vi "啮合 位移量对应扭矩.vi"(7 "目标位移量":dbl=136.0 format="%#_13g", 9 "扭矩":dbl[](array[numeric]), 11 "位移量":dbl[](array[numeric])) -> (3 "推力右扭矩":dbl)   [LabVIEW 2015, in "Logging.lvlib"]
uses:
  Logging.lvlib
panel:
  out "波形图 2":dbl[](graph)
  out "波形图":dbl[](graph)
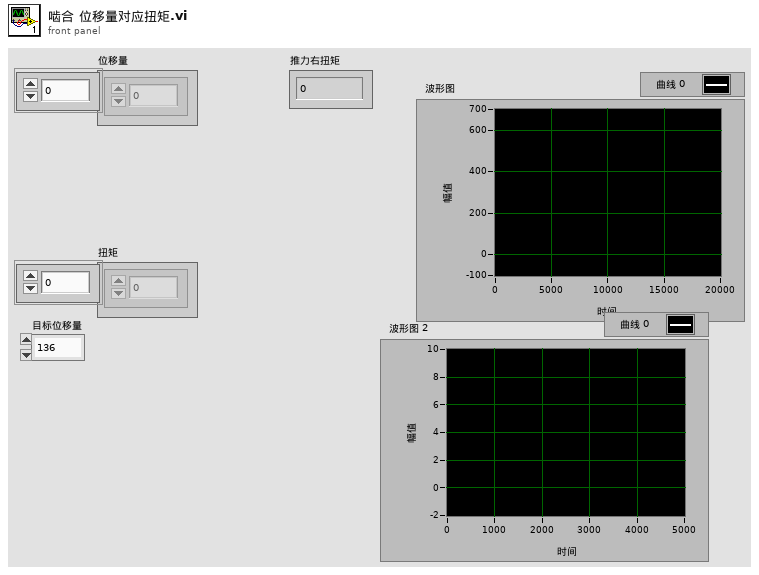
[diagram p1: front panel]
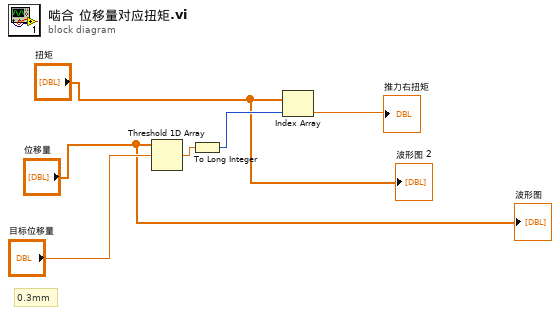
[diagram p0: block diagram]
diagram:
  # "0.3mm"
  n1 = Threshold 1D Array(2:"目标位移量", 3:"位移量") -> (0:w5:dbl)  [unwired: 1 in]
  n2 = To Long Integer(number=w5) -> (32bit integer=w3:i32)
  n3 = Index Array(array="扭矩", index=w3) -> (element=→"推力右扭矩":dbl)
  "波形图" <- "位移量"
  "波形图 2" <- "扭矩"
